vi "PinTest.vi"() -> ()   [LabVIEW 2012]
uses:
  Type/_RW Status.ctl
  <vilib>/Platform/TimedLoop/XDataNode/timing_clust.ctl
  <vilib>/Platform/TimedLoop/XDataNode/nitl_modes.ctl
  <vilib>/Platform/TimedLoop/XDataNode/wakeup.ctl
  <vilib>/rvi/Emulation/niFpgaSctlEmulationRegisterWithScheduler.vi
  <vilib>/rvi/Emulation/niFpgaSctlEmulationScheduler.vi
  <vilib>/rvi/Emulation/niFpgaSctlEmulationGetInTimedLoop.vi
  <vilib>/rvi/DataTransferAndStorage/Container/Common/niFpgaContainerGetUniqueNameForEmu.vi
  <vilib>/rvi/Memory/Memory_Emulation/niFpgaMemoryEmulationCacheClearOnFirstRun.vi
  <vilib>/rvi/Memory/Memory_Emulation/nirvimemoryEmulationManagerCache_MakeExclusive.vi
  <vilib>/rvi/Memory/Memory_Emulation/niFpgaMemoryEmulationValidateCache.vi
  <vilib>/rvi/Memory/Memory_Emulation/nirvimemoryEmulationManagerCache_ReleaseExclusive.vi
  <vilib>/rvi/Memory/Memory_Emulation/nirvimemoryEmulationManagerCache_InsertValue.vi
  <vilib>/Utility/error.llb/Clear Errors.vi
  <vilib>/rvi/Memory/Memory_Emulation/nirvimemoryEmulationManagerCache_GetValue.vi
  <vilib>/rvi/Emulation/niFpgaSctlEmulationGlobalWrite.vi
  <vilib>/rvi/Memory/Memory_Emulation/nirvimemoryEmulationManagerCache_SetValue.vi
  <vilib>/rvi/Emulation/niFpgaSctlEmulationResourceMgr.vi
  <vilib>/rvi/eio/common/nirviEmuTemplateMethod_errors.vi
  <vilib>/Platform/TimedLoop/XDataNode/XDataNode.xnode
  <vilib>/rvi/DataTransferAndStorage/Container/XNode/niFpgaContainer.xnode
  <vilib>/rvi/Memory/Memory_Emulation/nirvimemoryEmulation.vi
  <vilib>/eio/EIONode/EIONode.xnode
  <vilib>/Platform/TimedLoop/XDataNode/XDNodeRunTimeDep.lvlib
panel:
  in  "Address":u16
  in  "Data":u32
  in  "Read/Write 2":bool
  in  "RW Status":T1
  out "Version":u32=900130925
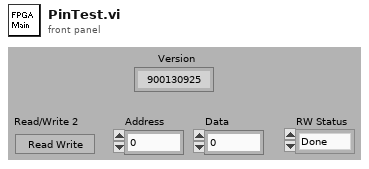
[diagram p1: front panel]
types:
  T1 = typedef "_RW Status.ctl" = enum8{"Done", "Do Read", "Do Write", "Set Latch1", "Set Latch2", "Set Latch3", "Set Latch4", "RP ON", "EL ON", "Serial Send", "Set LC Out", "Get LC In", "Read VAC", "Table Test", "Get Interlock", "Do Read2", "Do Write2"}
  T2 = typedef "XDNodeRunTimeDep.lvlib/timing_clust.ctl" = cluster{"Expected End [f-1]":u64, "Actual End [f-1]":u64, "Finished Late? [f-1]":bool, "Expected End [i-1]":u64, "Actual End [i-1]":u64, "Finished Late? [i-1]":bool, "Expected Start [i]":u64, "Actual Start [i]":u64, "Expected Start [f]":u64, "Actual Start [f]":u64, "Source Name":string, "Structure Name":string, "Period":i64, "Deadline":i64, "Offset":i64, "Start":i64, "Priority":i32, "Timeout":i32, "Mode":T3, "Wakeup Reason":T4, "Error":errorcluster, "Source Type":string, "Secondary Source Type":string, "Global End Time":u64, "Global Start Time":u64, "Frame Duration":u64, "Iteration Duration":u64, "Assigned CPU":i32, "I/O Scan Engine Mode":u32}
  T3 = typedef "XDNodeRunTimeDep.lvlib/nitl_modes.ctl" = enum32{"No Change", "Process missed periods, maintain original phase", "Discard missed periods, maintain original phase", "Process missed periods, ignore original phase", "Discard missed periods, ignore original phase"}
  T4 = typedef "XDNodeRunTimeDep.lvlib/wakeup.ctl" = enum32{"Normal", "Aborted", "Asynchronous wakeup", "Timing source error", "Timed loop error", "Timeout"}
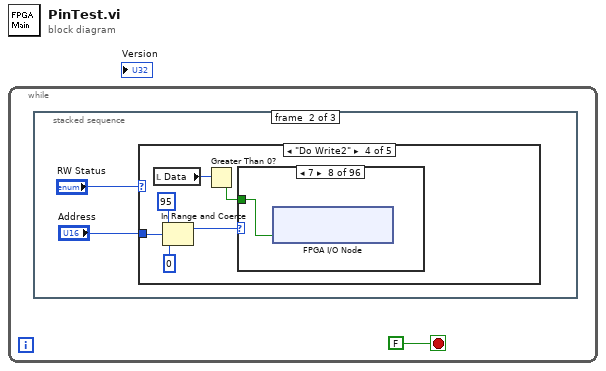
[diagram p0: block diagram]
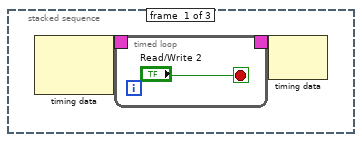
[diagram p2: hidden frame]
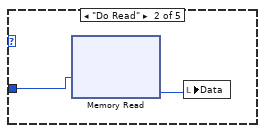
[diagram p4: hidden frame]
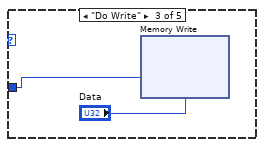
[diagram p5: hidden frame]
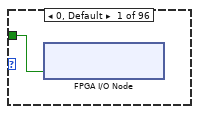
[diagram p6: hidden frame]
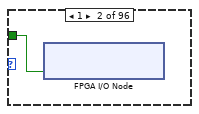
[diagram p7: hidden frame]
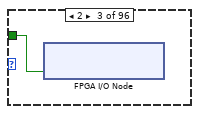
[diagram p8: hidden frame]
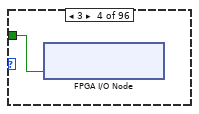
[diagram p9: hidden frame]
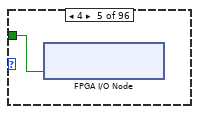
[diagram p10: hidden frame]
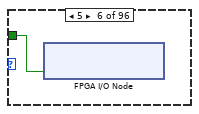
[diagram p11: hidden frame]
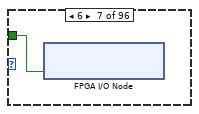
[diagram p12: hidden frame]
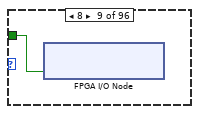
[diagram p13: hidden frame]
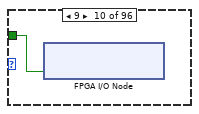
[diagram p14: hidden frame]
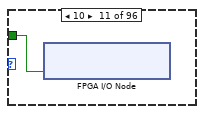
[diagram p15: hidden frame]
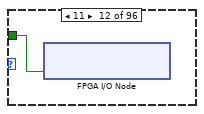
[diagram p16: hidden frame]
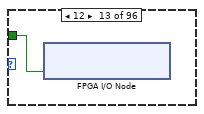
[diagram p17: hidden frame]
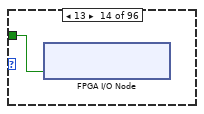
[diagram p18: hidden frame]
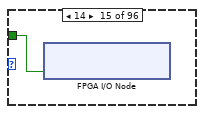
[diagram p19: hidden frame]
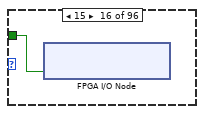
[diagram p20: hidden frame]
diagram:
  n1 = while {
    stop <- FALSE stop-if-true
    n2 = stacked-sequence {
      frame #0 {
        n3 = node-c288() -> (w3:T2)  [unwired: 2 in]
        n4 = timed-loop {
          timing-out: [_] -> w2
          timing: w3 -> [_]
          stop <- "Read/Write 2" stop-if-true
        }
        n5 = node-c288(w2) -> ()  [unwired: 1 out]
      }
      frame #1 {
        n6 = case shown="\"Do Write2\"" "RW Status" {
          tunnel: "Address" -> [_ w12 w14 w20 w122]
          frame "Done", Default {
          }
          frame "Do Read" {
            n7 = xnode ("Memory Read")("Address"=w12) -> ("Data"=w11:u32)  [unwired: 1 in, 1 out]
            n8 = local write "Data"(w11) -> ()
          }
          frame "Do Write" {
            n9 = xnode ("Memory Write")("Address"=w14, "Data"="Data") -> ()  [unwired: 1 in, 1 out]
          }
          frame "Do Write2" {
            n10 = local read "Data"() -> (w17:u32)
            n11 = In Range and Coerce(upper limit=u16 95, x=w20, lower limit=u16 0) -> (coerced(x)=w16:u16)  [unwired: 1 out]
            n12 = Greater Than 0?(x=w17) -> (x > 0?=w15:bool)
            n13 = case shown="7" w16 {
              tunnel: w15 -> [w21 w22 w23 w24 w25 w26 w27 w28 w29 w30 w31 w32 w33 w34 w35 w36 w37 w38 w39 w40 w41 w42 w43 w44 w45 w46 w47 w48 w49 w50 w51 w52 w53 w54 w55 w56 w57 w58 w59 w60 w61 w62 w63 w64 w65 w66 w67 w68 w69 w70 w71 w72 w73 w74 w75 w76 w77 w78 w79 w80 w81 w82 w83 w84 w85 w86 w87 w88 w89 w90 w91 w92 w93 w94 w95 w96 w97 w98 w99 w100 w101 w102 w103 w104 w105 w106 w107 w108 w109 w110 w111 w112 w113 w114 w115 w116]
              frame 0, Default {
                n14 = xnode "FPGA I/O Node"("Digtal IO/DIO0"=w21) -> ()  [unwired: 1 in, 1 out]
              }
              frame 1 {
                n15 = xnode "FPGA I/O Node"("Digtal IO/DIO1"=w22) -> ()  [unwired: 1 in, 1 out]
              }
              frame 2 {
                n16 = xnode "FPGA I/O Node"("Digtal IO/DIO2"=w23) -> ()  [unwired: 1 in, 1 out]
              }
              frame 3 {
                n17 = xnode "FPGA I/O Node"("Digtal IO/DIO3"=w24) -> ()  [unwired: 1 in, 1 out]
              }
              frame 4 {
                n18 = xnode "FPGA I/O Node"("Digtal IO/DIO4"=w25) -> ()  [unwired: 1 in, 1 out]
              }
              frame 5 {
                n19 = xnode "FPGA I/O Node"("Digtal IO/DIO5"=w26) -> ()  [unwired: 1 in, 1 out]
              }
              frame 6 {
                n20 = xnode "FPGA I/O Node"("Digtal IO/DIO6"=w27) -> ()  [unwired: 1 in, 1 out]
              }
              frame 7 {
                n21 = xnode "FPGA I/O Node"("Digtal IO/DIO7"=w28) -> ()  [unwired: 1 in, 1 out]
              }
              frame 8 {
                n22 = xnode "FPGA I/O Node"("Digtal IO/DIO8"=w29) -> ()  [unwired: 1 in, 1 out]
              }
              frame 9 {
                n23 = xnode "FPGA I/O Node"("Digtal IO/DIO9"=w30) -> ()  [unwired: 1 in, 1 out]
              }
              frame 10 {
                n24 = xnode "FPGA I/O Node"("Digtal IO/DIO10"=w31) -> ()  [unwired: 1 in, 1 out]
              }
              frame 11 {
                n25 = xnode "FPGA I/O Node"("Digtal IO/DIO11"=w32) -> ()  [unwired: 1 in, 1 out]
              }
              frame 12 {
                n26 = xnode "FPGA I/O Node"("Digtal IO/DIO12"=w33) -> ()  [unwired: 1 in, 1 out]
              }
              frame 13 {
                n27 = xnode "FPGA I/O Node"("Digtal IO/DIO13"=w34) -> ()  [unwired: 1 in, 1 out]
              }
              frame 14 {
                n28 = xnode "FPGA I/O Node"("Digtal IO/DIO14"=w35) -> ()  [unwired: 1 in, 1 out]
              }
              frame 15 {
                n29 = xnode "FPGA I/O Node"("Digtal IO/DIO15"=w36) -> ()  [unwired: 1 in, 1 out]
              }
              frame 16 {
                n30 = xnode "FPGA I/O Node"("Digtal IO/DIO16"=w37) -> ()  [unwired: 1 in, 1 out]
              }
              frame 17 {
                n31 = xnode "FPGA I/O Node"("Digtal IO/DIO17"=w38) -> ()  [unwired: 1 in, 1 out]
              }
              frame 18 {
                n32 = xnode "FPGA I/O Node"("Digtal IO/DIO18"=w39) -> ()  [unwired: 1 in, 1 out]
              }
              frame 19 {
                n33 = xnode "FPGA I/O Node"("Digtal IO/DIO19"=w40) -> ()  [unwired: 1 in, 1 out]
              }
              frame 20 {
                n34 = xnode "FPGA I/O Node"("Digtal IO/DIO20"=w41) -> ()  [unwired: 1 in, 1 out]
              }
              frame 21 {
                n35 = xnode "FPGA I/O Node"("Digtal IO/DIO21"=w42) -> ()  [unwired: 1 in, 1 out]
              }
              frame 22 {
                n36 = xnode "FPGA I/O Node"("Digtal IO/DIO22"=w43) -> ()  [unwired: 1 in, 1 out]
              }
              frame 23 {
                n37 = xnode "FPGA I/O Node"("Digtal IO/DIO23"=w44) -> ()  [unwired: 1 in, 1 out]
              }
              frame 24 {
                n38 = xnode "FPGA I/O Node"("Digtal IO/DIO24"=w45) -> ()  [unwired: 1 in, 1 out]
              }
              frame 25 {
                n39 = xnode "FPGA I/O Node"("Digtal IO/DIO25"=w46) -> ()  [unwired: 1 in, 1 out]
              }
              frame 26 {
                n40 = xnode "FPGA I/O Node"("Digtal IO/DIO26"=w47) -> ()  [unwired: 1 in, 1 out]
              }
              frame 27 {
                n41 = xnode "FPGA I/O Node"("Digtal IO/DIO27"=w48) -> ()  [unwired: 1 in, 1 out]
              }
              frame 28 {
                n42 = xnode "FPGA I/O Node"("Digtal IO/DIO28"=w49) -> ()  [unwired: 1 in, 1 out]
              }
              frame 29 {
                n43 = xnode "FPGA I/O Node"("Digtal IO/DIO29"=w50) -> ()  [unwired: 1 in, 1 out]
              }
              frame 30 {
                n44 = xnode "FPGA I/O Node"("Digtal IO/DIO30"=w51) -> ()  [unwired: 1 in, 1 out]
              }
              frame 31 {
                n45 = xnode "FPGA I/O Node"("Digtal IO/DIO31"=w52) -> ()  [unwired: 1 in, 1 out]
              }
              frame 32 {
                n46 = xnode "FPGA I/O Node"("Digtal IO/DIO32"=w53) -> ()  [unwired: 1 in, 1 out]
              }
              frame 33 {
                n47 = xnode "FPGA I/O Node"("Digtal IO/DIO33"=w54) -> ()  [unwired: 1 in, 1 out]
              }
              frame 34 {
                n48 = xnode "FPGA I/O Node"("Digtal IO/DIO34"=w55) -> ()  [unwired: 1 in, 1 out]
              }
              frame 35 {
                n49 = xnode "FPGA I/O Node"("Digtal IO/DIO35"=w56) -> ()  [unwired: 1 in, 1 out]
              }
              frame 36 {
                n50 = xnode "FPGA I/O Node"("Digtal IO/DIO36"=w57) -> ()  [unwired: 1 in, 1 out]
              }
              frame 37 {
                n51 = xnode "FPGA I/O Node"("Digtal IO/DIO37"=w58) -> ()  [unwired: 1 in, 1 out]
              }
              frame 38 {
                n52 = xnode "FPGA I/O Node"("Digtal IO/DIO38"=w59) -> ()  [unwired: 1 in, 1 out]
              }
              frame 39 {
                n53 = xnode "FPGA I/O Node"("Digtal IO/DIO39"=w60) -> ()  [unwired: 1 in, 1 out]
              }
              frame 40 {
                n54 = xnode "FPGA I/O Node"("Digtal IO/DIO40"=w61) -> ()  [unwired: 1 in, 1 out]
              }
              frame 41 {
                n55 = xnode "FPGA I/O Node"("Digtal IO/DIO41"=w62) -> ()  [unwired: 1 in, 1 out]
              }
              frame 42 {
                n56 = xnode "FPGA I/O Node"("Digtal IO/DIO42"=w63) -> ()  [unwired: 1 in, 1 out]
              }
              frame 43 {
                n57 = xnode "FPGA I/O Node"("Digtal IO/DIO43"=w64) -> ()  [unwired: 1 in, 1 out]
              }
              frame 44 {
                n58 = xnode "FPGA I/O Node"("Digtal IO/DIO44"=w65) -> ()  [unwired: 1 in, 1 out]
              }
              frame 45 {
                n59 = xnode "FPGA I/O Node"("Digtal IO/DIO45"=w66) -> ()  [unwired: 1 in, 1 out]
              }
              frame 46 {
                n60 = xnode "FPGA I/O Node"("Digtal IO/DIO46"=w67) -> ()  [unwired: 1 in, 1 out]
              }
              frame 47 {
                n61 = xnode "FPGA I/O Node"("Digtal IO/DIO47"=w68) -> ()  [unwired: 1 in, 1 out]
              }
              frame 48 {
                n62 = xnode "FPGA I/O Node"("Digtal IO/DIO48"=w69) -> ()  [unwired: 1 in, 1 out]
              }
              frame 49 {
                n63 = xnode "FPGA I/O Node"("Digtal IO/DIO49"=w70) -> ()  [unwired: 1 in, 1 out]
              }
              frame 50 {
                n64 = xnode "FPGA I/O Node"("Digtal IO/DIO50"=w71) -> ()  [unwired: 1 in, 1 out]
              }
              frame 51 {
                n65 = xnode "FPGA I/O Node"("Digtal IO/DIO51"=w72) -> ()  [unwired: 1 in, 1 out]
              }
              frame 52 {
                n66 = xnode "FPGA I/O Node"("Digtal IO/DIO52"=w73) -> ()  [unwired: 1 in, 1 out]
              }
              frame 53 {
                n67 = xnode "FPGA I/O Node"("Digtal IO/DIO53"=w74) -> ()  [unwired: 1 in, 1 out]
              }
              frame 54 {
                n68 = xnode "FPGA I/O Node"("Digtal IO/DIO54"=w75) -> ()  [unwired: 1 in, 1 out]
              }
              frame 55 {
                n69 = xnode "FPGA I/O Node"("Digtal IO/DIO55"=w76) -> ()  [unwired: 1 in, 1 out]
              }
              frame 56 {
                n70 = xnode "FPGA I/O Node"("Digtal IO/DIO56"=w77) -> ()  [unwired: 1 in, 1 out]
              }
              frame 57 {
                n71 = xnode "FPGA I/O Node"("Digtal IO/DIO57"=w78) -> ()  [unwired: 1 in, 1 out]
              }
              frame 58 {
                n72 = xnode "FPGA I/O Node"("Digtal IO/DIO58"=w79) -> ()  [unwired: 1 in, 1 out]
              }
              frame 59 {
                n73 = xnode "FPGA I/O Node"("Digtal IO/DIO59"=w80) -> ()  [unwired: 1 in, 1 out]
              }
              frame 60 {
                n74 = xnode "FPGA I/O Node"("Digtal IO/DIO60"=w81) -> ()  [unwired: 1 in, 1 out]
              }
              frame 61 {
                n75 = xnode "FPGA I/O Node"("Digtal IO/DIO61"=w82) -> ()  [unwired: 1 in, 1 out]
              }
              frame 62 {
                n76 = xnode "FPGA I/O Node"("Digtal IO/DIO62"=w83) -> ()  [unwired: 1 in, 1 out]
              }
              frame 63 {
                n77 = xnode "FPGA I/O Node"("Digtal IO/DIO63"=w84) -> ()  [unwired: 1 in, 1 out]
              }
              frame 64 {
                n78 = xnode "FPGA I/O Node"("Digtal IO/DIO64"=w85) -> ()  [unwired: 1 in, 1 out]
              }
              frame 65 {
                n79 = xnode "FPGA I/O Node"("Digtal IO/DIO65"=w86) -> ()  [unwired: 1 in, 1 out]
              }
              frame 66 {
                n80 = xnode "FPGA I/O Node"("Digtal IO/DIO66"=w87) -> ()  [unwired: 1 in, 1 out]
              }
              frame 67 {
                n81 = xnode "FPGA I/O Node"("Digtal IO/DIO67"=w88) -> ()  [unwired: 1 in, 1 out]
              }
              frame 68 {
                n82 = xnode "FPGA I/O Node"("Digtal IO/DIO68"=w89) -> ()  [unwired: 1 in, 1 out]
              }
              frame 69 {
                n83 = xnode "FPGA I/O Node"("Digtal IO/DIO69"=w90) -> ()  [unwired: 1 in, 1 out]
              }
              frame 70 {
                n84 = xnode "FPGA I/O Node"("Digtal IO/DIO70"=w91) -> ()  [unwired: 1 in, 1 out]
              }
              frame 71 {
                n85 = xnode "FPGA I/O Node"("Digtal IO/DIO71"=w92) -> ()  [unwired: 1 in, 1 out]
              }
              frame 72 {
                n86 = xnode "FPGA I/O Node"("Digtal IO/DIO72"=w93) -> ()  [unwired: 1 in, 1 out]
              }
              frame 73 {
                n87 = xnode "FPGA I/O Node"("Digtal IO/DIO73"=w94) -> ()  [unwired: 1 in, 1 out]
              }
              frame 74 {
                n88 = xnode "FPGA I/O Node"("Digtal IO/DIO74"=w95) -> ()  [unwired: 1 in, 1 out]
              }
              frame 75 {
                n89 = xnode "FPGA I/O Node"("Digtal IO/DIO75"=w96) -> ()  [unwired: 1 in, 1 out]
              }
              frame 76 {
                n90 = xnode "FPGA I/O Node"("Digtal IO/DIO76"=w97) -> ()  [unwired: 1 in, 1 out]
              }
              frame 77 {
                n91 = xnode "FPGA I/O Node"("Digtal IO/DIO77"=w98) -> ()  [unwired: 1 in, 1 out]
              }
              frame 78 {
                n92 = xnode "FPGA I/O Node"("Digtal IO/DIO78"=w99) -> ()  [unwired: 1 in, 1 out]
              }
              frame 79 {
                n93 = xnode "FPGA I/O Node"("Digtal IO/DIO79"=w100) -> ()  [unwired: 1 in, 1 out]
              }
              frame 80 {
                n94 = xnode "FPGA I/O Node"("Digtal IO/DIO80"=w101) -> ()  [unwired: 1 in, 1 out]
              }
              frame 81 {
                n95 = xnode "FPGA I/O Node"("Digtal IO/DIO81"=w102) -> ()  [unwired: 1 in, 1 out]
              }
              frame 82 {
                n96 = xnode "FPGA I/O Node"("Digtal IO/DIO82"=w103) -> ()  [unwired: 1 in, 1 out]
              }
              frame 83 {
                n97 = xnode "FPGA I/O Node"("Digtal IO/DIO83"=w104) -> ()  [unwired: 1 in, 1 out]
              }
              frame 84 {
                n98 = xnode "FPGA I/O Node"("Digtal IO/DIO84"=w105) -> ()  [unwired: 1 in, 1 out]
              }
              frame 85 {
                n99 = xnode "FPGA I/O Node"("Digtal IO/DIO85"=w106) -> ()  [unwired: 1 in, 1 out]
              }
              frame 86 {
                n100 = xnode "FPGA I/O Node"("Digtal IO/DIO86"=w107) -> ()  [unwired: 1 in, 1 out]
              }
              frame 87 {
                n101 = xnode "FPGA I/O Node"("Digtal IO/DIO87"=w108) -> ()  [unwired: 1 in, 1 out]
              }
              frame 88 {
                n102 = xnode "FPGA I/O Node"("Digtal IO/DIO88"=w109) -> ()  [unwired: 1 in, 1 out]
              }
              frame 89 {
                n103 = xnode "FPGA I/O Node"("Digtal IO/DIO89"=w110) -> ()  [unwired: 1 in, 1 out]
              }
              frame 90 {
                n104 = xnode "FPGA I/O Node"("Digtal IO/DIO90"=w111) -> ()  [unwired: 1 in, 1 out]
              }
              frame 91 {
                n105 = xnode "FPGA I/O Node"("Digtal IO/DIO91"=w112) -> ()  [unwired: 1 in, 1 out]
              }
              frame 92 {
                n106 = xnode "FPGA I/O Node"("Digtal IO/DIO92"=w113) -> ()  [unwired: 1 in, 1 out]
              }
              frame 93 {
                n107 = xnode "FPGA I/O Node"("Digtal IO/DIO93"=w114) -> ()  [unwired: 1 in, 1 out]
              }
              frame 94 {
                n108 = xnode "FPGA I/O Node"("Digtal IO/DIO94"=w115) -> ()  [unwired: 1 in, 1 out]
              }
              frame 95 {
                n109 = xnode "FPGA I/O Node"("Digtal IO/DIO95"=w116) -> ()  [unwired: 1 in, 1 out]
              }
            }
          }
          frame "Do Read2" {
            n110 = In Range and Coerce(upper limit=u16 95, x=w122, lower limit=u16 0) -> (coerced(x)=w119:u16)  [unwired: 1 out]
            n111 = case shown="2" w119 {
              tunnel: [w123 w124 w125 w126 w127 w128 w129 w130 w131 w132 w133 w134 w135 w136 w137 w138 w139 w140 w141 w142 w143 w144 w145 w146 w147 w148 w149 w150 w151 w152 w153 w154 w155 w156 w157 w158 w159 w160 w161 w162 w163 w164 w165 w166 w167 w168 w169 w170 w171 w172 w173 w174 w175 w176 w177 w178 w179 w180 w181 w182 w183 w184 w185 w186 w187 w188 w189 w190 w191 w192 w193 w194 w195 w196 w197 w198 w199 w200 w201 w202 w203 w204 w205 w206 w207 w208 w209 w210 w211 w212 w213 w214 w215 w216 w217 w218] -> w118
              frame 0, Default {
                n112 = xnode "FPGA I/O Node"() -> ("Digtal IO/DIO0"=w123:bool)  [unwired: 1 in, 1 out]
              }
              frame 1 {
                n113 = xnode "FPGA I/O Node"() -> ("Digtal IO/DIO0"=w124:bool)  [unwired: 1 in, 1 out]
              }
              frame 2 {
                n114 = xnode "FPGA I/O Node"() -> ("Digtal IO/DIO2"=w125:bool)  [unwired: 1 in, 1 out]
              }
              frame 3 {
                n115 = xnode "FPGA I/O Node"() -> ("Digtal IO/DIO3"=w126:bool)  [unwired: 1 in, 1 out]
              }
              frame 4 {
                n116 = xnode "FPGA I/O Node"() -> ("Digtal IO/DIO4"=w127:bool)  [unwired: 1 in, 1 out]
              }
              frame 5 {
                n117 = xnode "FPGA I/O Node"() -> ("Digtal IO/DIO5"=w128:bool)  [unwired: 1 in, 1 out]
              }
              frame 6 {
                n118 = xnode "FPGA I/O Node"() -> ("Digtal IO/DIO6"=w129:bool)  [unwired: 1 in, 1 out]
              }
              frame 7 {
                n119 = xnode "FPGA I/O Node"() -> ("Digtal IO/DIO7"=w130:bool)  [unwired: 1 in, 1 out]
              }
              frame 8 {
                n120 = xnode "FPGA I/O Node"() -> ("Digtal IO/DIO8"=w131:bool)  [unwired: 1 in, 1 out]
              }
              frame 9 {
                n121 = xnode "FPGA I/O Node"() -> ("Digtal IO/DIO9"=w132:bool)  [unwired: 1 in, 1 out]
              }
              frame 10 {
                n122 = xnode "FPGA I/O Node"() -> ("Digtal IO/DIO10"=w133:bool)  [unwired: 1 in, 1 out]
              }
              frame 11 {
                n123 = xnode "FPGA I/O Node"() -> ("Digtal IO/DIO11"=w134:bool)  [unwired: 1 in, 1 out]
              }
              frame 12 {
                n124 = xnode "FPGA I/O Node"() -> ("Digtal IO/DIO12"=w135:bool)  [unwired: 1 in, 1 out]
              }
              frame 13 {
                n125 = xnode "FPGA I/O Node"() -> ("Digtal IO/DIO13"=w136:bool)  [unwired: 1 in, 1 out]
              }
              frame 14 {
                n126 = xnode "FPGA I/O Node"() -> ("Digtal IO/DIO14"=w137:bool)  [unwired: 1 in, 1 out]
              }
              frame 15 {
                n127 = xnode "FPGA I/O Node"() -> ("Digtal IO/DIO15"=w138:bool)  [unwired: 1 in, 1 out]
              }
              frame 16 {
                n128 = xnode "FPGA I/O Node"() -> ("Digtal IO/DIO16"=w139:bool)  [unwired: 1 in, 1 out]
              }
              frame 17 {
                n129 = xnode "FPGA I/O Node"() -> ("Digtal IO/DIO17"=w140:bool)  [unwired: 1 in, 1 out]
              }
              frame 18 {
                n130 = xnode "FPGA I/O Node"() -> ("Digtal IO/DIO18"=w141:bool)  [unwired: 1 in, 1 out]
              }
              frame 19 {
                n131 = xnode "FPGA I/O Node"() -> ("Digtal IO/DIO19"=w142:bool)  [unwired: 1 in, 1 out]
              }
              frame 20 {
                n132 = xnode "FPGA I/O Node"() -> ("Digtal IO/DIO20"=w143:bool)  [unwired: 1 in, 1 out]
              }
              frame 21 {
                n133 = xnode "FPGA I/O Node"() -> ("Digtal IO/DIO21"=w144:bool)  [unwired: 1 in, 1 out]
              }
              frame 22 {
                n134 = xnode "FPGA I/O Node"() -> ("Digtal IO/DIO22"=w145:bool)  [unwired: 1 in, 1 out]
              }
              frame 23 {
                n135 = xnode "FPGA I/O Node"() -> ("Digtal IO/DIO23"=w146:bool)  [unwired: 1 in, 1 out]
              }
              frame 24 {
                n136 = xnode "FPGA I/O Node"() -> ("Digtal IO/DIO24"=w147:bool)  [unwired: 1 in, 1 out]
              }
              frame 25 {
                n137 = xnode "FPGA I/O Node"() -> ("Digtal IO/DIO25"=w148:bool)  [unwired: 1 in, 1 out]
              }
              frame 26 {
                n138 = xnode "FPGA I/O Node"() -> ("Digtal IO/DIO26"=w149:bool)  [unwired: 1 in, 1 out]
              }
              frame 27 {
                n139 = xnode "FPGA I/O Node"() -> ("Digtal IO/DIO27"=w150:bool)  [unwired: 1 in, 1 out]
              }
              frame 28 {
                n140 = xnode "FPGA I/O Node"() -> ("Digtal IO/DIO28"=w151:bool)  [unwired: 1 in, 1 out]
              }
              frame 29 {
                n141 = xnode "FPGA I/O Node"() -> ("Digtal IO/DIO29"=w152:bool)  [unwired: 1 in, 1 out]
              }
              frame 30 {
                n142 = xnode "FPGA I/O Node"() -> ("Digtal IO/DIO30"=w153:bool)  [unwired: 1 in, 1 out]
              }
              frame 31 {
                n143 = xnode "FPGA I/O Node"() -> ("Digtal IO/DIO31"=w154:bool)  [unwired: 1 in, 1 out]
              }
              frame 32 {
                n144 = xnode "FPGA I/O Node"() -> ("Digtal IO/DIO32"=w155:bool)  [unwired: 1 in, 1 out]
              }
              frame 33 {
                n145 = xnode "FPGA I/O Node"() -> ("Digtal IO/DIO33"=w156:bool)  [unwired: 1 in, 1 out]
              }
              frame 34 {
                n146 = xnode "FPGA I/O Node"() -> ("Digtal IO/DIO34"=w157:bool)  [unwired: 1 in, 1 out]
              }
              frame 35 {
                n147 = xnode "FPGA I/O Node"() -> ("Digtal IO/DIO35"=w158:bool)  [unwired: 1 in, 1 out]
              }
              frame 36 {
                n148 = xnode "FPGA I/O Node"() -> ("Digtal IO/DIO36"=w159:bool)  [unwired: 1 in, 1 out]
              }
              frame 37 {
                n149 = xnode "FPGA I/O Node"() -> ("Digtal IO/DIO37"=w160:bool)  [unwired: 1 in, 1 out]
              }
              frame 38 {
                n150 = xnode "FPGA I/O Node"() -> ("Digtal IO/DIO38"=w161:bool)  [unwired: 1 in, 1 out]
              }
              frame 39 {
                n151 = xnode "FPGA I/O Node"() -> ("Digtal IO/DIO39"=w162:bool)  [unwired: 1 in, 1 out]
              }
              frame 40 {
                n152 = xnode "FPGA I/O Node"() -> ("Digtal IO/DIO40"=w163:bool)  [unwired: 1 in, 1 out]
              }
              frame 41 {
                n153 = xnode "FPGA I/O Node"() -> ("Digtal IO/DIO41"=w164:bool)  [unwired: 1 in, 1 out]
              }
              frame 42 {
                n154 = xnode "FPGA I/O Node"() -> ("Digtal IO/DIO42"=w165:bool)  [unwired: 1 in, 1 out]
              }
              frame 43 {
                n155 = xnode "FPGA I/O Node"() -> ("Digtal IO/DIO43"=w166:bool)  [unwired: 1 in, 1 out]
              }
              frame 44 {
                n156 = xnode "FPGA I/O Node"() -> ("Digtal IO/DIO44"=w167:bool)  [unwired: 1 in, 1 out]
              }
              frame 45 {
                n157 = xnode "FPGA I/O Node"() -> ("Digtal IO/DIO45"=w168:bool)  [unwired: 1 in, 1 out]
              }
              frame 46 {
                n158 = xnode "FPGA I/O Node"() -> ("Digtal IO/DIO46"=w169:bool)  [unwired: 1 in, 1 out]
              }
              frame 47 {
                n159 = xnode "FPGA I/O Node"() -> ("Digtal IO/DIO47"=w170:bool)  [unwired: 1 in, 1 out]
              }
              frame 48 {
                n160 = xnode "FPGA I/O Node"() -> ("Digtal IO/DIO48"=w171:bool)  [unwired: 1 in, 1 out]
              }
              frame 49 {
                n161 = xnode "FPGA I/O Node"() -> ("Digtal IO/DIO49"=w172:bool)  [unwired: 1 in, 1 out]
              }
              frame 50 {
                n162 = xnode "FPGA I/O Node"() -> ("Digtal IO/DIO50"=w173:bool)  [unwired: 1 in, 1 out]
              }
              frame 51 {
                n163 = xnode "FPGA I/O Node"() -> ("Digtal IO/DIO51"=w174:bool)  [unwired: 1 in, 1 out]
              }
              frame 52 {
                n164 = xnode "FPGA I/O Node"() -> ("Digtal IO/DIO52"=w175:bool)  [unwired: 1 in, 1 out]
              }
              frame 53 {
                n165 = xnode "FPGA I/O Node"() -> ("Digtal IO/DIO53"=w176:bool)  [unwired: 1 in, 1 out]
              }
              frame 54 {
                n166 = xnode "FPGA I/O Node"() -> ("Digtal IO/DIO54"=w177:bool)  [unwired: 1 in, 1 out]
              }
              frame 55 {
                n167 = xnode "FPGA I/O Node"() -> ("Digtal IO/DIO55"=w178:bool)  [unwired: 1 in, 1 out]
              }
              frame 56 {
                n168 = xnode "FPGA I/O Node"() -> ("Digtal IO/DIO56"=w179:bool)  [unwired: 1 in, 1 out]
              }
              frame 57 {
                n169 = xnode "FPGA I/O Node"() -> ("Digtal IO/DIO57"=w180:bool)  [unwired: 1 in, 1 out]
              }
              frame 58 {
                n170 = xnode "FPGA I/O Node"() -> ("Digtal IO/DIO58"=w181:bool)  [unwired: 1 in, 1 out]
              }
              frame 59 {
                n171 = xnode "FPGA I/O Node"() -> ("Digtal IO/DIO59"=w182:bool)  [unwired: 1 in, 1 out]
              }
              frame 60 {
                n172 = xnode "FPGA I/O Node"() -> ("Digtal IO/DIO60"=w183:bool)  [unwired: 1 in, 1 out]
              }
              frame 61 {
                n173 = xnode "FPGA I/O Node"() -> ("Digtal IO/DIO61"=w184:bool)  [unwired: 1 in, 1 out]
              }
              frame 62 {
                n174 = xnode "FPGA I/O Node"() -> ("Digtal IO/DIO62"=w185:bool)  [unwired: 1 in, 1 out]
              }
              frame 63 {
                n175 = xnode "FPGA I/O Node"() -> ("Digtal IO/DIO63"=w186:bool)  [unwired: 1 in, 1 out]
              }
              frame 64 {
                n176 = xnode "FPGA I/O Node"() -> ("Digtal IO/DIO64"=w187:bool)  [unwired: 1 in, 1 out]
              }
              frame 65 {
                n177 = xnode "FPGA I/O Node"() -> ("Digtal IO/DIO65"=w188:bool)  [unwired: 1 in, 1 out]
              }
              frame 66 {
                n178 = xnode "FPGA I/O Node"() -> ("Digtal IO/DIO66"=w189:bool)  [unwired: 1 in, 1 out]
              }
              frame 67 {
                n179 = xnode "FPGA I/O Node"() -> ("Digtal IO/DIO67"=w190:bool)  [unwired: 1 in, 1 out]
              }
              frame 68 {
                n180 = xnode "FPGA I/O Node"() -> ("Digtal IO/DIO68"=w191:bool)  [unwired: 1 in, 1 out]
              }
              frame 69 {
                n181 = xnode "FPGA I/O Node"() -> ("Digtal IO/DIO69"=w192:bool)  [unwired: 1 in, 1 out]
              }
              frame 70 {
                n182 = xnode "FPGA I/O Node"() -> ("Digtal IO/DIO70"=w193:bool)  [unwired: 1 in, 1 out]
              }
              frame 71 {
                n183 = xnode "FPGA I/O Node"() -> ("Digtal IO/DIO71"=w194:bool)  [unwired: 1 in, 1 out]
              }
              frame 72 {
                n184 = xnode "FPGA I/O Node"() -> ("Digtal IO/DIO72"=w195:bool)  [unwired: 1 in, 1 out]
              }
              frame 73 {
                n185 = xnode "FPGA I/O Node"() -> ("Digtal IO/DIO73"=w196:bool)  [unwired: 1 in, 1 out]
              }
              frame 74 {
                n186 = xnode "FPGA I/O Node"() -> ("Digtal IO/DIO74"=w197:bool)  [unwired: 1 in, 1 out]
              }
              frame 75 {
                n187 = xnode "FPGA I/O Node"() -> ("Digtal IO/DIO75"=w198:bool)  [unwired: 1 in, 1 out]
              }
              frame 76 {
                n188 = xnode "FPGA I/O Node"() -> ("Digtal IO/DIO76"=w199:bool)  [unwired: 1 in, 1 out]
              }
              frame 77 {
                n189 = xnode "FPGA I/O Node"() -> ("Digtal IO/DIO77"=w200:bool)  [unwired: 1 in, 1 out]
              }
              frame 78 {
                n190 = xnode "FPGA I/O Node"() -> ("Digtal IO/DIO78"=w201:bool)  [unwired: 1 in, 1 out]
              }
              frame 79 {
                n191 = xnode "FPGA I/O Node"() -> ("Digtal IO/DIO79"=w202:bool)  [unwired: 1 in, 1 out]
              }
              frame 80 {
                n192 = xnode "FPGA I/O Node"() -> ("Digtal IO/DIO80"=w203:bool)  [unwired: 1 in, 1 out]
              }
              frame 81 {
                n193 = xnode "FPGA I/O Node"() -> ("Digtal IO/DIO81"=w204:bool)  [unwired: 1 in, 1 out]
              }
              frame 82 {
                n194 = xnode "FPGA I/O Node"() -> ("Digtal IO/DIO82"=w205:bool)  [unwired: 1 in, 1 out]
              }
              frame 83 {
                n195 = xnode "FPGA I/O Node"() -> ("Digtal IO/DIO83"=w206:bool)  [unwired: 1 in, 1 out]
              }
              frame 84 {
                n196 = xnode "FPGA I/O Node"() -> ("Digtal IO/DIO84"=w207:bool)  [unwired: 1 in, 1 out]
              }
              frame 85 {
                n197 = xnode "FPGA I/O Node"() -> ("Digtal IO/DIO85"=w208:bool)  [unwired: 1 in, 1 out]
              }
              frame 86 {
                n198 = xnode "FPGA I/O Node"() -> ("Digtal IO/DIO86"=w209:bool)  [unwired: 1 in, 1 out]
              }
              frame 87 {
                n199 = xnode "FPGA I/O Node"() -> ("Digtal IO/DIO87"=w210:bool)  [unwired: 1 in, 1 out]
              }
              frame 88 {
                n200 = xnode "FPGA I/O Node"() -> ("Digtal IO/DIO88"=w211:bool)  [unwired: 1 in, 1 out]
              }
              frame 89 {
                n201 = xnode "FPGA I/O Node"() -> ("Digtal IO/DIO89"=w212:bool)  [unwired: 1 in, 1 out]
              }
              frame 90 {
                n202 = xnode "FPGA I/O Node"() -> ("Digtal IO/DIO90"=w213:bool)  [unwired: 1 in, 1 out]
              }
              frame 91 {
                n203 = xnode "FPGA I/O Node"() -> ("Digtal IO/DIO91"=w214:bool)  [unwired: 1 in, 1 out]
              }
              frame 92 {
                n204 = xnode "FPGA I/O Node"() -> ("Digtal IO/DIO92"=w215:bool)  [unwired: 1 in, 1 out]
              }
              frame 93 {
                n205 = xnode "FPGA I/O Node"() -> ("Digtal IO/DIO93"=w216:bool)  [unwired: 1 in, 1 out]
              }
              frame 94 {
                n206 = xnode "FPGA I/O Node"() -> ("Digtal IO/DIO94"=w217:bool)  [unwired: 1 in, 1 out]
              }
              frame 95 {
                n207 = xnode "FPGA I/O Node"() -> ("Digtal IO/DIO95"=w218:bool)  [unwired: 1 in, 1 out]
              }
            }
            n208 = Boolean To (0,1)(Boolean=w118) -> (0, 1=w117:i16)
            n209 = local write "Data"(w117) -> ()
          }
        }
      }
      frame #2 {
        n210 = local write "RW Status"(_RW_Status."Done" ("RW Status")) -> ()
      }
    }
  }
